vi "Wait Chart.vi"() -> ()   [LabVIEW 2009]
doc: "Ce VI est un exercice du cours LabVIEW Fondamental 1.\n\nIl est utilisé pour expliquer les différences entre les fonctions Attendre et Temps écoulé."
uses:
  Instance           1 18Saved   Wait Chart .vi
panel:
  out "Temps écoulé":dbl(graph)
  out "Fonction Attendre":dbl(graph)
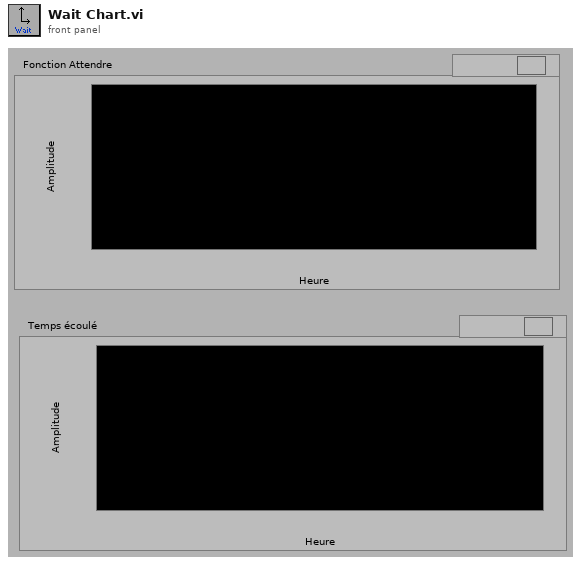
[diagram p1: front panel]
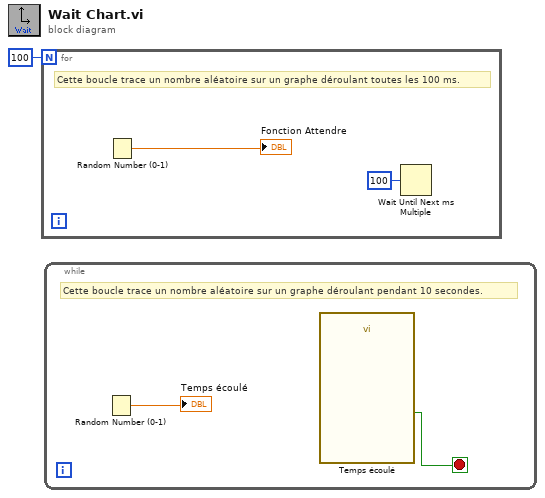
[diagram p0: block diagram]
diagram:
  n1 = for "Boucle For" {
    N: 100 -> [_]
    # "Cette boucle trace un nombre aléatoire sur un graphe déroulant toutes les 100 ms."
    n2 = Random Number (0-1) ("Nombre aléatoire (0-1)")() -> (number: 0 to 1=→"Fonction Attendre":dbl)
    n3 = Wait Until Next ms Multiple ("Attendre un multiple de ms")(millisecond multiple=u32 100) -> ()  [unwired: 1 out]
  }
  n4 = while "Boucle While" {
    stop <- w4 stop-if-true
    # "Cette boucle trace un nombre aléatoire sur un graphe déroulant pendant 10 secondes."
    n5 = Random Number (0-1) ("Nombre aléatoire (0-1)")() -> (number: 0 to 1=→"Temps écoulé":dbl)
    n6 = call "Temps écoulé"() -> ("Time has Elapsed"=w4:bool)  [unwired: 5 in, 14 out]
  }
